vi "Analyze.vi"(0 "Analyze Q-Factor in":refnum<class "Analyze q-Factor.lvclass">, 1 "Create Overlay?":bool, 5 "Image in":T1, 7 "Parameters":variant, 9 "Results in":variant, 11 "error in (no error)":errorcluster) -> (4 "Analyze Q-Factor out":refnum<class "Analyze q-Factor.lvclass">, 6 "Image out":T1, 8 "Parameters out":variant, 10 "Results":variant, 15 "error out":errorcluster)   [LabVIEW 2020, in "Analyze.lvlib" / "Analyze q-Factor.lvclass"]
uses:
  Analyze q-Factor.lvclass
  <vilib>/vision/Image Controls.llb/IMAQ Image.ctl
  Analyze Fluence/Fluence Info.ctl
  Width Method.ctl
  Analyze BaseClass/Analyze BaseClass.lvclass
  Analyze Fluence/Analyze Fluence.lvclass
  <vilib>/vision/NI_Vision_Development_Module.lvlib
panel:
  in  "Energy  A4 or A5 [J]":dbl=10.0
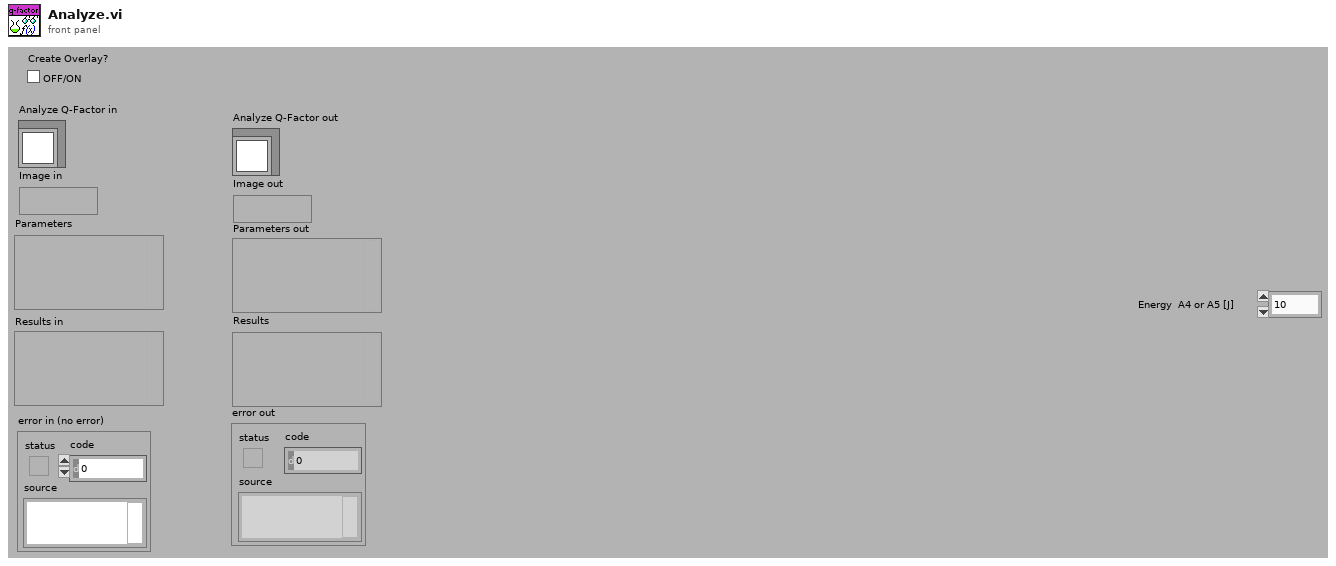
[diagram p1: front panel]
types:
  T1 = typedef "IMAQ Image.ctl" = refnum<image>
  T2 = typedef "Width Method.ctl" = enum16{"FWHM", "1/e", "1/e^2", "80%", "90%"}
  T3 = typedef "Image Type" = u32
  T4 = typedef "Analyze.lvlib/Analyze Fluence.lvclass/Fluence Info.ctl" = cluster{"Fluence J/cm^2":dbl, "Energy in Area":dbl, "max value":i64, "Max fluence area":cluster{"Left":i32, "Top":i32, "Right":i32, "Bottom":i32}}
  T5 = typedef "ROI Descriptor" = cluster{"Global Rectangle":i32[], "Contours":cluster{"ID":enum32{"External", "Internal"}, "Type":u32, "Coordinates":i32[]}[]}
  T6 = cluster{"Mean Value":sgl, "Standard Variation":sgl, "Minimal Value":sgl, "Maximal Value":sgl, "Area (calibrated)":sgl, "Area (pixels)":i32, "%":sgl}
  T7 = cluster{"Left":i32, "Top":i32, "Right":i32, "Bottom":i32, sgl}
  T8 = cluster{"Desired Font (Application)":enum16{"User-specified Font", "Application Font", "System Font", "Dialog Font"}, "[User-specified Font]":cluster{"Font Name":string, "Size":i16, "Strikeout?":bool, "Italic?":bool, "Underline?":bool, "Outline?":bool, "Shadow?":bool, "Bold?":bool, "Rotation Angle":dbl}, "Horizontal Alignment":i16, "Vertical Alignment":i16}
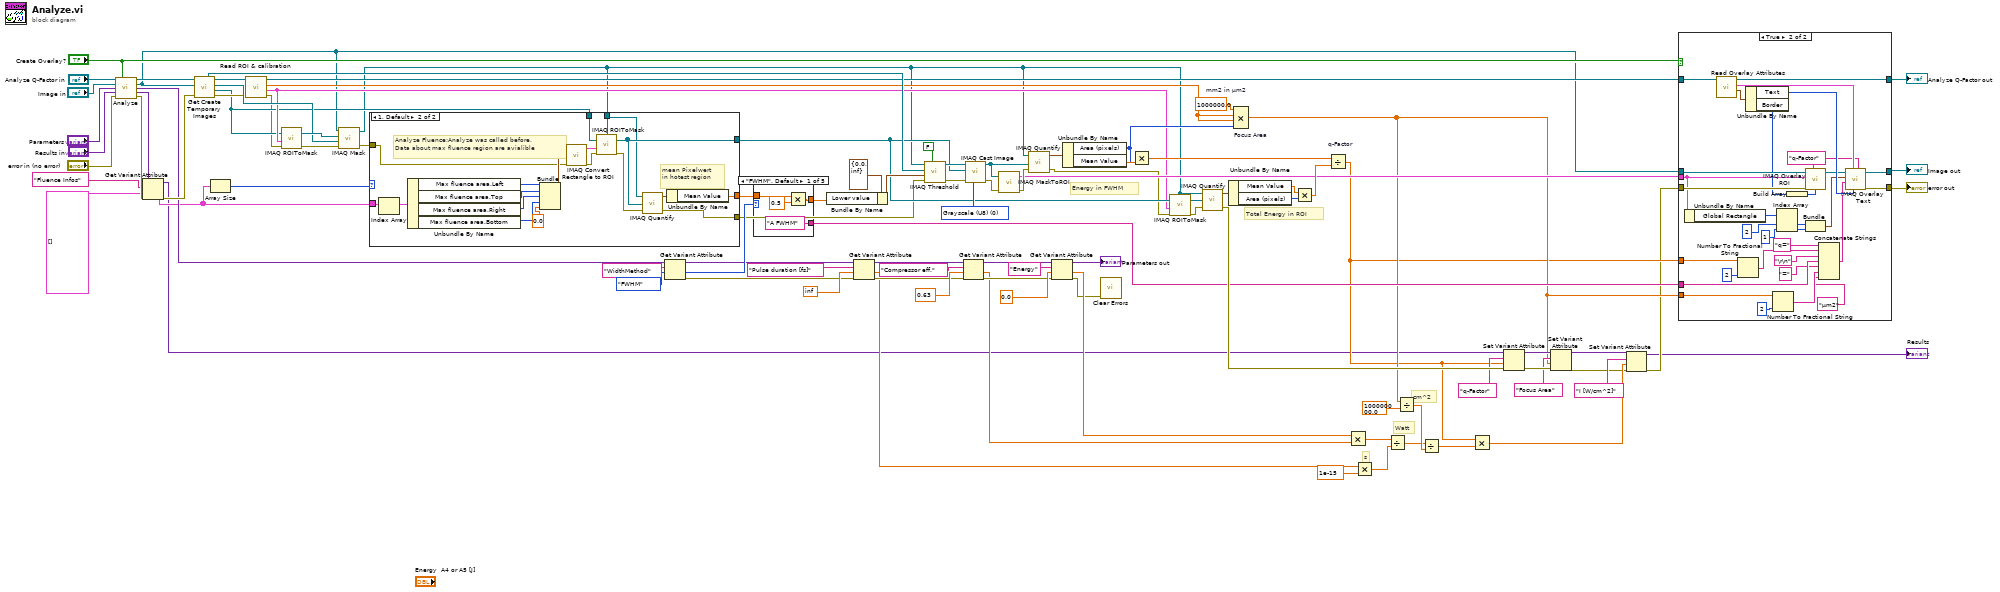
[diagram p0: block diagram]
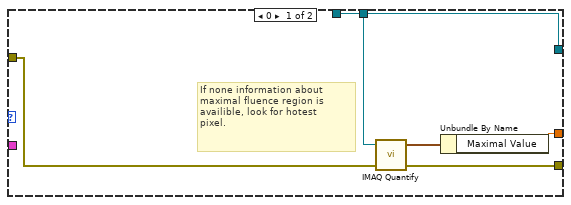
[diagram p2: hidden frame]
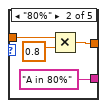
[diagram p4: hidden frame]
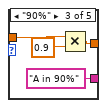
[diagram p5: hidden frame]
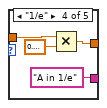
[diagram p6: hidden frame]
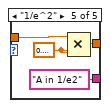
[diagram p7: hidden frame]
diagram:
  w34 = 1000000.0  # mm2 in µm2
  w84 = T3 0 items=["Grayscale (U8)", "Grayscale (I16)", "Grayscale (SGL)", "Complex (CSG)", "RGB (U32)", "HSL (U32)", "RGB (U64)", "Grayscale (U16)"] ("Image Type")
  # "cm^2"
  # "s"
  # "Watt"
  # "Total Energy in ROI"
  # "Energy in FWHM"
  n1 = call-parent "Analyze.vi"("Analyze BaseClass in"="Analyze Q-Factor in", "Create Overlay?"="Create Overlay?", "Image in"="Image in", "Parameters"="Parameters", "Results in"="Results in", "error in (no error)"="error in (no error)") -> ("Analyze BaseClass out"=w91:refnum<class "Analyze q-Factor.lvclass">, "Image out"=w35:T1, "Parameters out"=w73:variant, "Results"=w92:variant, "error out"=w95:errorcluster)  [unwired: 5 in]
  n2 = Get Variant Attribute(Variant=w92, name="Fluence Infos", default value (empty Variant)=T4[] [], error in=w95) -> (duplicate Variant=w11:variant, value=w48:T4[], error out=w90:errorcluster)  [unwired: 1 out]
  n3 = call-dynamic "Get Create Temporary Images.vi"("error in (no error)"=w90, "Image in"=w35, "Analyze BaseClass in"=w91) -> ("error out"=w41:errorcluster, "image mask"=w39:T1, "work image"=w43:T1, "Analyze BaseClass out"=w82:refnum<class "Analyze q-Factor.lvclass">, "masked image"=w87:T1)  [unwired: 4 in]
  n4 = Array Size(array=w48) -> (size(s)=w49:i32)
  n5 = call-dynamic "Read ROI & calibration.vi"("error in (no error)"=w41, "Analyze BaseClass in"=w82) -> ("error out"=w38:errorcluster, "ROI Descriptor"=w40:T5, "calibration mm/px"=w66:dbl, "Analyze BaseClass out"=w64:refnum<class "Analyze q-Factor.lvclass">)  [unwired: 6 in]
  n6 = call "IMAQ ROIToMask"("error in (no error)"=w38, "ROI Descriptor"=w40, "Image"=w39) -> ("error out"=w44:errorcluster, "Image Out"=w45:T1)  [unwired: 3 in, 1 out]
  n7 = call "IMAQ Mask"("error in (no error)"=w44, "Image Dst"=w43, "Image Mask"=w45, "Image Src"=w35) -> ("error out"=w37:errorcluster, "Image Dst Out"=w36:T1)  [unwired: 1 in]
  n8 = case shown="1, Default" w49 {
    tunnel: w48 -> [_ w124]
    tunnel: w37 -> [w104 w118]
    tunnel: w39 -> [w105 w117]
    tunnel: [w105 w116] -> w53
    tunnel: [w103 w113] -> w52
    tunnel: [w102 w112] -> w51
    tunnel: w36 -> [w101 w107]
    frame 0 {
      # "If none information about \nmaximal fluence region is\navailible, look for hotest\npixel."
      n9 = call "IMAQ Quantify"("error in (no error)"=w104, "Image"=w101) -> ("error out"=w103:errorcluster, "Global Report"=w106:T6)  [unwired: 1 in, 1 out]
      n10 = Unbundle By Name(w106) -> ("Maximal Value"=w102:sgl)
    }
    frame 1, Default {
      # "Analyze Fluence:Analyze was called before,\nData about max fluence region are avialible"
      # "mean Pixelwert\nin hotest region"
      n11 = Index Array(array=w124) -> (element=w123:T4)  [unwired: 1 in]
      n12 = Unbundle By Name(w123) -> ("Max fluence area.Left"=w111:i32, "Max fluence area.Top"=w110:i32, "Max fluence area.Right"=w109:i32, "Max fluence area.Bottom"=w108:i32)
      n13 = Bundle("Left"=w111, "Top"=w110, "Right"=w109, "Bottom"=w108, sgl 0.0) -> (w121:T7)  [unwired: 1 in]
      n14 = call "IMAQ Convert Rectangle to ROI"("error in (no error)"=w118, "Rectangle"=w121) -> ("error out"=w119:errorcluster, "ROI Descriptor"=w120:T5)  [unwired: 7 in]
      n15 = call "IMAQ ROIToMask"("error in (no error)"=w119, "ROI Descriptor"=w120, "Image"=w117, "Image Model"=w107) -> ("error out"=w115:errorcluster, "Image Out"=w116:T1)  [unwired: 2 in, 1 out]
      n16 = call "IMAQ Quantify"("error in (no error)"=w115, "Image Mask"=w116, "Image"=w107) -> ("error out"=w113:errorcluster, "Global Report"=w114:T6)  [unwired: 1 out]
      n17 = Unbundle By Name(w114) -> ("Mean Value"=w112:sgl)
    }
  }
  n18 = Get Variant Attribute(Variant=w73, name="WidthMethod", default value (empty Variant)=Width_Method."FWHM" ("Methode")) -> (duplicate Variant=w10:variant, value=w70:T2, error out=w8:errorcluster)  [unwired: 1 in, 1 out]
  n19 = case shown="\"FWHM\", Default" w70 {
    tunnel: w51 -> [w127 w131 w135 w139 w144]
    tunnel: [w126 w130 w134 w138 w143] -> w69
    tunnel: ["A FWHM" "A in 80%" "A in 90%" "A in 1/e" "A in 1/e2"] -> w47
    frame "FWHM", Default {
      n20 = Multiply(x=w127, y=0.5) -> (x*y=w126:dbl)
    }
    frame "80%" {
      n21 = Multiply(x=w131, y=0.8) -> (x*y=w130:dbl)
    }
    frame "90%" {
      n22 = Multiply(x=w135, y=0.9) -> (x*y=w134:dbl)
    }
    frame "1/e" {
      n23 = Multiply(x=w139, y=0.36787944117144233) -> (x*y=w138:dbl)
    }
    frame "1/e^2" {
      w142 = 0.36787944117144233
      n24 = Compound Arithmetic op=MULTIPLY(w144, w142, w142) -> (w143:dbl)
    }
  }
  n25 = Bundle By Name(cluster=cluster{"Lower value":sgl, "Upper value":sgl} {"Lower value"=0.0, "Upper value"=inf} ("Range"), "Lower value"=w69) -> (w88:cluster{"Lower value":sgl, "Upper value":sgl})
  n26 = Get Variant Attribute(Variant=w10, name="Pulse duration [fs]", default value (empty Variant)=inf, error in=w8) -> (duplicate Variant=w31:variant, value=w16:dbl, error out=w25:errorcluster)  [unwired: 1 out]
  n27 = call "IMAQ Threshold"("Keep/Replace Value (Replace)"=FALSE, "error in (no error)"=w52, "Range"=w88, "Image Dst"=w87, "Image Src"=w36) -> ("error out"=w85:errorcluster, "Image Dst Out"=w86:T1)  [unwired: 5 in]
  n28 = Get Variant Attribute(Variant=w31, name="Compressor eff.", default value (empty Variant)=0.63, error in=w25) -> (duplicate Variant=w28:variant, value=w12:dbl, error out=w24:errorcluster)  [unwired: 1 out]
  n29 = call "IMAQ Cast Image"("Image Type"=w84, "error in (no error)"=w85, "Image Dst"=w53, "Image Src"=w86) -> ("error out"=w56:errorcluster, "Image Dst Out"=w57:T1)  [unwired: 6 in]
  n30 = call "IMAQ MaskToROI"("Image"=w57, "error in (no error)"=w56) -> ("ROI Descriptor"=w54:T5, "error out"=w55:errorcluster)  [unwired: 5 in, 1 out]
  n31 = call "IMAQ Quantify"("error in (no error)"=w55, "Image Mask"=w57, "Image"=w36) -> ("error out"=w42:errorcluster, "Global Report"=w83:T6)  [unwired: 1 out]
  n32 = Get Variant Attribute(Variant=w28, name="Energy", default value (empty Variant)=0.0, error in=w24) -> (duplicate Variant=→"Parameters out":variant, value=w15:dbl, error out=w7:errorcluster)  [unwired: 1 out]
  n33 = Unbundle By Name(w83) -> ("Area (pixels)"=w58:i32, "Mean Value"=w65:sgl)
  n34 = call <vilib>:"Clear Errors.vi"("error in (no error)"=w7) -> ()  [unwired: 5 in, 2 out]
  n35 = Multiply(x=w65, y=w58) -> (x*y=w76:sgl)
  n36 = call "IMAQ ROIToMask"("error in (no error)"=w42, "ROI Descriptor"=w40, "Image"=w53, "Image Model"=w36) -> ("error out"=w75:errorcluster, "Image Out"=w78:T1)  [unwired: 2 in, 1 out]
  n37 = call "IMAQ Quantify"("error in (no error)"=w75, "Image Mask"=w78, "Image"=w36) -> ("error out"=w74:errorcluster, "Global Report"=w79:T6)  [unwired: 1 out]
  n38 = Unbundle By Name(w79) -> ("Mean Value"=w81:sgl, "Area (pixels)"=w80:i32)
  n39 = Compound Arithmetic op=MULTIPLY "Focus Area"(w34, w66, w66, w58) -> (w14:dbl)
  n40 = Multiply(x=w81, y=w80) -> (x*y=w77:sgl)
  n41 = Divide "q-Factor"(x=w76, y=w77) -> (x/y=w13:sgl)
  n42 = Multiply(x=w15, y=w12) -> (x*y=w17:dbl)
  n43 = Multiply(x=w16, y=1e-15) -> (x*y=w18:dbl)
  n44 = Divide(x=w17, y=w18) -> (x/y=w20:dbl)
  n45 = Divide(x=w14, y=100000000.0) -> (x/y=w22:dbl)
  n46 = Divide(x=w20, y=w22) -> (x/y=w23:dbl)
  n47 = Multiply(x=w13, y=w23) -> (x*y=w4:dbl)
  n48 = Set Variant Attribute(Variant=w11, name="q-Factor", value=w13, error in=w74) -> (Variant out=w68:variant, error out=w67:errorcluster)  [unwired: 1 out]
  n49 = Set Variant Attribute(Variant=w68, name="Focus Area", value=w14, error in=w67) -> (Variant out=w6:variant, error out=w3:errorcluster)  [unwired: 1 out]
  n50 = Set Variant Attribute(Variant=w6, name="I [W/cm^2]", value=w4, error in=w3) -> (Variant out=→"Results":variant, error out=w2:errorcluster)  [unwired: 1 out]
  n51 = case shown="True" "Create Overlay?" {
    tunnel: w35 -> [w147 w163]
    tunnel: [w147 w179] -> w61
    tunnel: w2 -> [w146 w161]
    tunnel: [w146 w178] -> w60
    tunnel: [w145 w176] -> w63
    tunnel: w64 -> [w145 w175]
    tunnel: w13 -> [_ w170]
    tunnel: w47 -> [_ w168]
    tunnel: w54 -> [_ w155]
    tunnel: w14 -> [_ w148]
    frame False {
    }
    frame True {
      w158 = "q-Factor" ("name")
      n52 = Unbundle By Name(w155) -> ("Global Rectangle"=w152:i32[])
      n53 = call-dynamic "Read Overlay Attributes.vi"("Analyze BaseClass in"=w175) -> ("Overlay colors"=w174:cluster{"Border":u32, "Text":u32}, "Font, Size & Style"=w173:T8, "Analyze BaseClass out"=w176:refnum<class "Analyze q-Factor.lvclass">)  [unwired: 7 in, 1 out]
      n54 = Number To Fractional String(number=w170, precision (6)=i16 2) -> (F-format string=w169:string)  [unwired: 2 in]
      n55 = Unbundle By Name(w174) -> ("Text"=w177:u32, "Border"=w160:u32)
      n56 = Number To Fractional String(number=w148, precision (6)=i16 2) -> (F-format string=w164:string)  [unwired: 2 in]
      n57 = Index Array(array=w152, index #1=2 ("index"), index #2=1 ("index")) -> (element #1=w154:i32, element #2=w153:i32)
      n58 = Build Array(w160) -> (w159:u32[])
      n59 = call "IMAQ Overlay ROI"("Colors (Green)"=w159, "Group"=w158, "error in (no error)"=w161, "ROI Descriptor"=w155, "Image"=w163) -> ("Image Out"=w162:T1)  [unwired: 5 in, 1 out]
      n60 = Bundle(w154, w153) -> (w172:cluster{i32, i32})  [unwired: 1 in]
      n61 = Concatenate Strings("q=" ("name"), w169, "\r\n", w168, "=" ("string"), w164, "µm2" ("string")) -> (w171:string)
      n62 = call "IMAQ Overlay Text"("Group"=w158, "Text Color (black)"=w177, "Font, Size & Style"=w173, "String"=w171, "Origin"=w172, "Image"=w162) -> ("error out"=w178:errorcluster, "Image Out"=w179:T1)  [unwired: 4 in]
    }
  }
  "error out" <- w60
  "Analyze Q-Factor out" <- w63
  "Image out" <- w61
